vi "Calibration.vi"() -> ()   [LabVIEW 2015]
uses:
  <vilib>/DAQmx/read.llb/DAQmx Read (Analog 1D Wfm NChan 1Samp).vi
  <vilib>/DAQmx/read.llb/DAQmx Read (Analog Wfm 1Chan 1Samp).vi
  <vilib>/DAQmx/miscellaneous.llb/DAQmx Fill In Error Info.vi
panel:
  out "Salvando?":bool
  in  "Enable":bool=TRUE
  in  "Filename":string
  out "RTD Temperature":waveform(dbl)(graph)
  out "Iteration":i32
  out "Shunt - Current":dbl(knob) scale=0.0..30.0
  out "Total":dbl(knob) scale=0.0..30.0
  out "Gray-Orange Resistor":dbl(knob) scale=0.0..30.0
  out "Orange-Red Resistor":dbl(knob) scale=0.0..30.0
  in  "stop 3":bool
  out "Red-Gray Resistor":dbl(knob) scale=0.0..30.0
  in  "stop":bool
  out "RTD":dbl(slide) scale=0.0..100.0
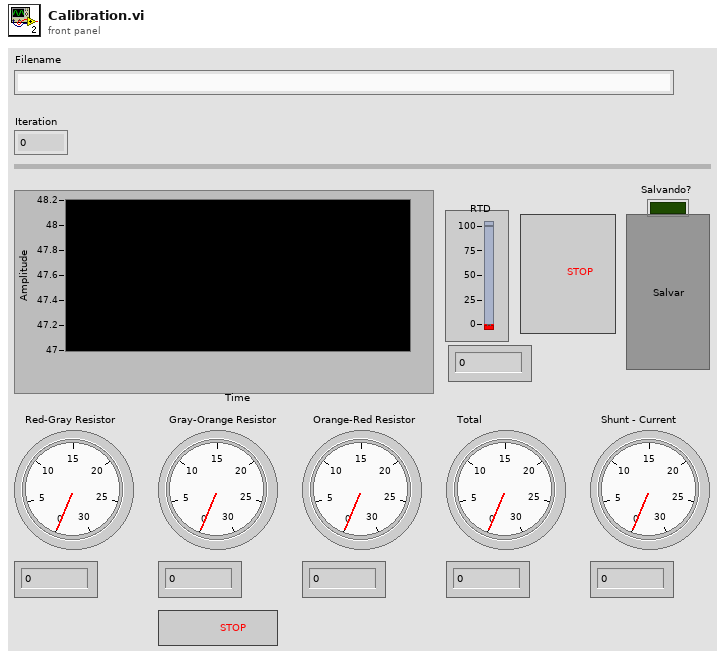
[diagram p1: front panel]
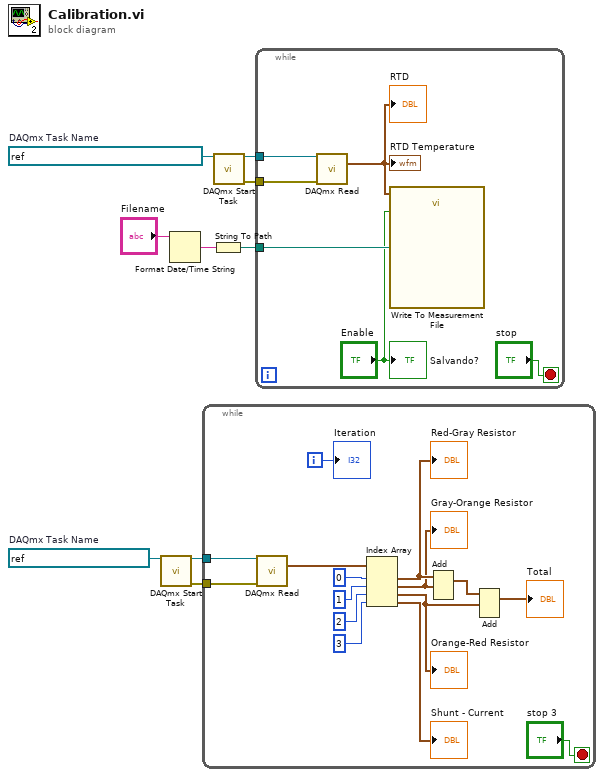
[diagram p0: block diagram]
diagram:
  w4 = refnum<k21> "Voltage Reading Task"  # DAQmx Task Name
  w9 = refnum<k21> "RTD Temperature Reading Task"  # DAQmx Task Name
  n1 = call <vilib>:"DAQmx Start Task.vi"("task/channels in"=w4) -> ("task out"=w6:refnum<k21>, "error out"=w5:errorcluster)  [unwired: 13 in]
  n2 = Format Date/Time String(time format string (%c)="Filename") -> (date/time string=w2:string)  [unwired: 2 in]
  n3 = while {
    tunnel: w6 -> [w23]
    tunnel: w5 -> [w22]
    i -> [w12]
    stop <- "stop 3" stop-if-true
    n4 = call-poly <vilib>:"DAQmx Read.vi"("task/channels in"=w23, "error in"=w22) -> ("data"=w10:waveform(dbl)[])  [unwired: 11 in, 2 out]
    n5 = Index Array(array=w10, index #1=0 ("index"), index #2=1 ("index"), index #3=2 ("index"), index #4=3 ("index")) -> (element #1=w18:waveform(dbl), element #2=w16:waveform(dbl), element #3=w14:waveform(dbl), element #4=→"Shunt - Current":waveform(dbl))
    "Red-Gray Resistor" <- w18
    "Orange-Red Resistor" <- w14
    "Gray-Orange Resistor" <- w16
    n6 = Add(1:w16, 2:w18) -> (0:w20:waveform(dbl))  [unwired: 1 in, 1 out]
    n7 = Add(1:w14, 2:w20) -> (0:→"Total":waveform(dbl))  [unwired: 1 in, 1 out]
    "Iteration" <- w12
  }
  n8 = String To Path(string=w2) -> (path=w1:path)
  n9 = call <vilib>:"DAQmx Start Task.vi"("task/channels in"=w9) -> ("task out"=w8:refnum<k21>, "error out"=w7:errorcluster)  [unwired: 13 in]
  n10 = while {
    tunnel: w8 -> [w29]
    tunnel: w7 -> [w28]
    tunnel: w1 -> [w27]
    stop <- "stop" stop-if-true
    n11 = call-poly <vilib>:"DAQmx Read.vi"("task/channels in"=w29, "error in"=w28) -> ("data"=w26:waveform(dbl))  [unwired: 11 in, 2 out]
    "RTD" <- w26
    "RTD Temperature" <- w26
    n12 = call "Write To Measurement File"("Signals"=w26, "Enable"="Enable", "Filename"=w27) -> ()  [unwired: 14 in, 3 out]
    "Salvando?" <- "Enable"
  }
